vi "LabviewDemo.vi"() -> ()   [LabVIEW 2023]
uses:
  vmmsolib/vmmsolib.lvlib
panel:
  out "Support Samples":u32[](array[numeric])
  out "InitDll Return":i32
  out "Device is OK?":i32
  out "FinishDll Return":i32
  out "Voltage Wave":dbl[](graph)
  out "Voltage Array":dbl[](array[numeric]) caption="采集电压数组"
  out "ReadVoltageData Return":u32
  in  "Stop":bool
  out "Capture Return":i32
  out "Sample Success？":i32
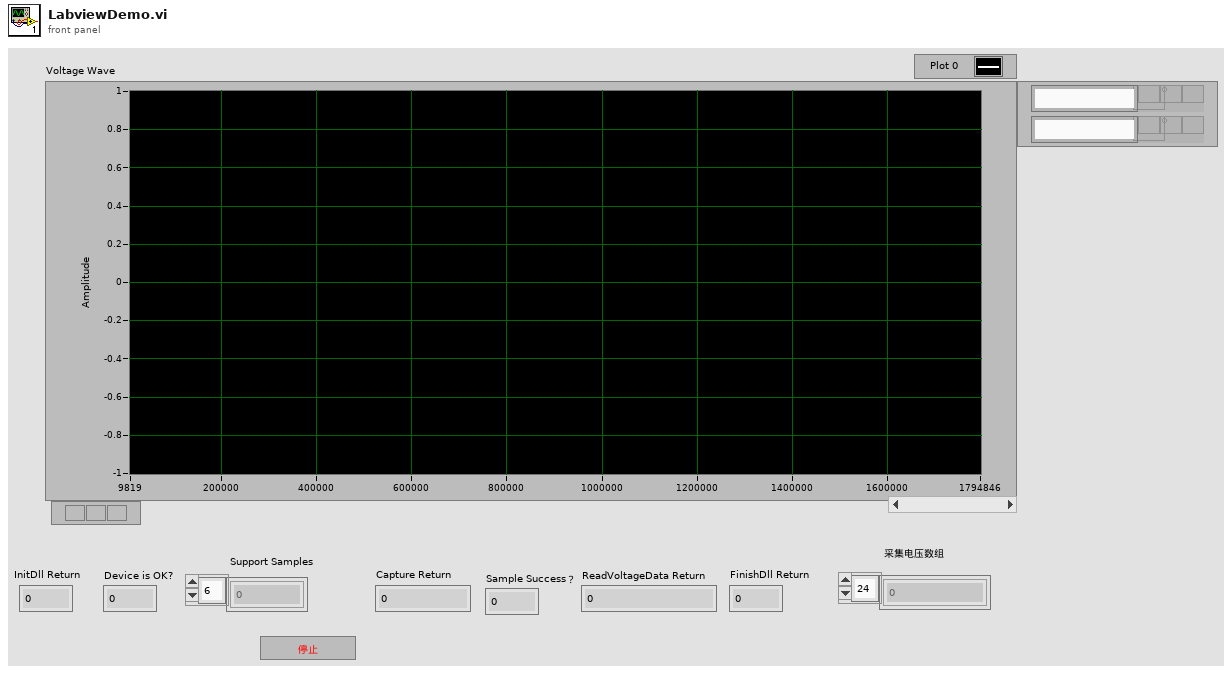
[diagram p1: front panel]
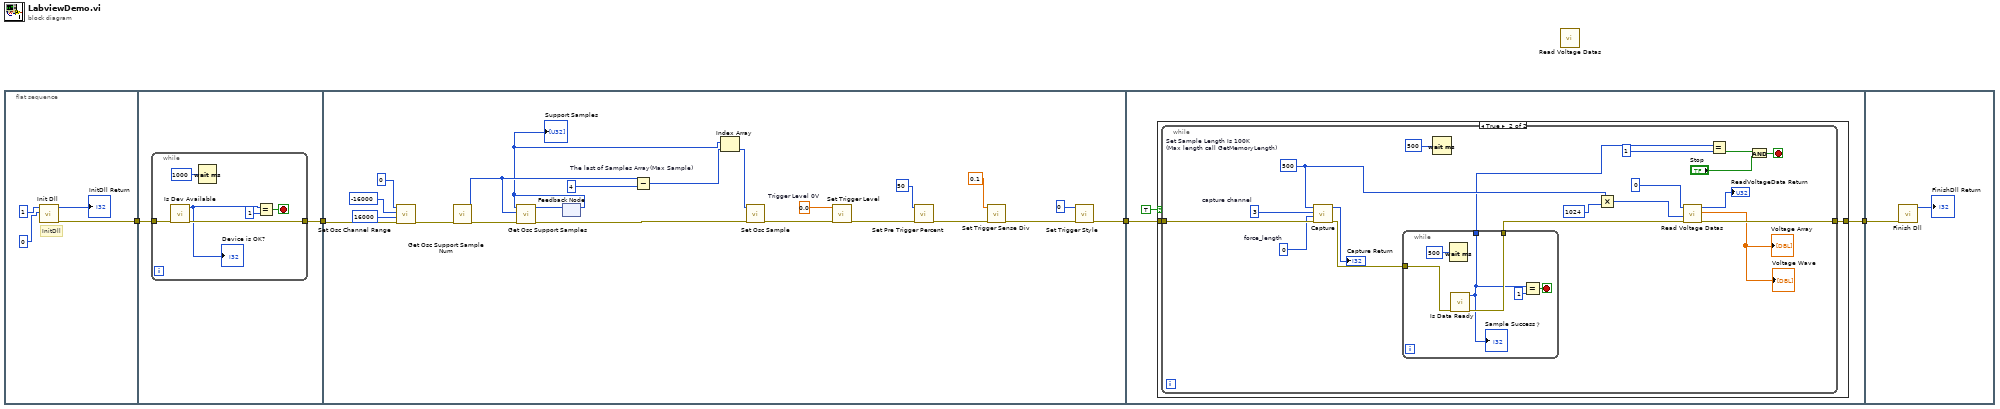
[diagram p0: block diagram]
diagram:
  n1 = flat-sequence {
    tunnel: [w8] -> w4
    tunnel: w4 -> [w10]
    tunnel: [w9] -> w3
    tunnel: w3 -> [w36]
    tunnel: [w28] -> w2
    tunnel: w2 -> [w41]
    tunnel: [w39] -> w1
    tunnel: w1 -> [w70]
    frame #0 {
      # "InitDll"
      n2 = call "Init Dll.vi"("en_hard_watchdog"=0 ("channel"), "en_log"=1 ("channel")) -> ("error out"=w8:errorcluster, "function return"=→"InitDll Return":i32)  [unwired: 8 in]
    }
    frame #1 {
      n3 = while {
        tunnel: w10 -> [w13]
        tunnel: [w12] -> w9
        stop <- w14 stop-if-true
        n4 = call "Is Dev Available.vi"("error in (no error)"=w13) -> ("error out"=w12:errorcluster, "function return"=w11:i32)  [unwired: 9 in]
        "Device is OK?" <- w11
        n5 = Wait (ms)(milliseconds to wait=u32 1000 ("等待时间（毫秒）")) -> ()  [unwired: 1 out]
        n6 = Equal?(x=w11, y=1) -> (x = y?=w14:bool)
      }
    }
    frame #2 {
      w26 = sgl 0.0  # Trigger Level 0V
      n7 = call "Set Osc Channel Range.vi"("error in (no error)"=w36, "maxmv"=16000 ("minmv"), "minmv"=-16000, "channel"=0) -> ("error out"=w25:errorcluster)  [unwired: 6 in, 1 out]
      n8 = call "Get Osc Support Sample Num.vi"("error in (no error)"=w25) -> ("error out"=w24:errorcluster, "function return"=w19:i32)  [unwired: 9 in]
      n9 = feedback #1() -> (w17:u32[])  [unwired: 1 in]
      "Support Samples" <- w17
      n10 = call "Get Osc Support Samples.vi"("error in (no error)"=w24, "maxnum"=w19, "sample"=w17) -> ("error out"=w23:errorcluster, "sample out"=w18:u32[])  [unwired: 6 in, 1 out]
      n11 = feedback-in #1(w18) -> ()
      n12 = Subtract "The last of Samples Array(Max Sample)"(x=w19, y=4 ("front")) -> (x-y=w21:i32)
      n13 = Index Array(array=w17, index=w21) -> (element=w22:u32)
      n14 = call "Set Osc Sample.vi"("error in (no error)"=w23, "sample"=w22) -> ("error out"=w33:errorcluster)  [unwired: 8 in, 1 out]
      n15 = call "Set Trigger Level.vi"("error in (no error)"=w33, "level"=w26) -> ("error out"=w31:errorcluster)  [unwired: 9 in]
      n16 = call "Set Pre Trigger Percent.vi"("error in (no error)"=w31, "front"=50) -> ("error out"=w30:errorcluster)  [unwired: 9 in]
      n17 = call "Set Trigger Sense Div.vi"("error in (no error)"=w30, "sense"=0.1) -> ("error out"=w29:errorcluster)  [unwired: 9 in]
      n18 = call "Set Trigger Style.vi"("error in (no error)"=w29, "style"=u32 0) -> ("error out"=w28:errorcluster)  [unwired: 9 in]
    }
    frame #3 {
      n19 = case shown="True" TRUE {
        tunnel: w41 -> [_ w42]
        tunnel: [_ w43] -> w39
        frame False {
        }
        frame True {
          n20 = while {
            tunnel: [w55] -> w43
            tunnel: w42 -> [w56]
            stop <- w59 stop-if-true
            w47 = i8 0  # force_length
            w52 = u32 500  # Set Sample Length Is 100K (Max length call GetMemoryLength)
            w48 = i8 3  # capture channel
            n21 = call "Capture.vi"("error in (no error)"=w56, "force_length"=w47, "capture_channel"=w48, "length"=w52) -> ("error out"=w46:errorcluster, "function return"=→"Capture Return":i32)  [unwired: 6 in]
            n22 = while {
              tunnel: w46 -> [w65]
              tunnel: [w64] -> w45
              tunnel: [w63] -> w44
              stop <- w66 stop-if-true
              n23 = Wait (ms)(milliseconds to wait=u32 500 ("等待时间（毫秒）")) -> ()  [unwired: 1 out]
              n24 = call "Is Data Ready.vi"("error in (no error)"=w65) -> ("error out"=w64:errorcluster, "function return"=w63:i32)  [unwired: 9 in]
              "Sample Success？" <- w63
              n25 = Equal?(x=w63, y=1) -> (x = y?=w66:bool)
            }
            n26 = Wait (ms)(milliseconds to wait=u32 500 ("等待时间（毫秒）")) -> ()  [unwired: 1 out]
            n27 = Multiply(x=w52, y=1024) -> (x*y=w51:u32)
            n28 = call "Read Voltage Datas.vi"("error in (no error)"=w45, "length"=w51, "channel"=i8 0) -> ("error out"=w55:errorcluster, "buffer out"=→"Voltage Array" →"Voltage Wave":dbl[], "function return"=→"ReadVoltageData Return":u32)  [unwired: 6 in]
            n29 = Equal?(x=w44, y=1) -> (x = y?=w57:bool)
            n30 = And(x=w57, y="Stop") -> (x .and. y?=w59:bool)
          }
        }
      }
    }
    frame #4 {
      n31 = call "Finish Dll.vi"("error in (no error)"=w70) -> ("function return"=→"FinishDll Return":i32)  [unwired: 9 in, 1 out]
    }
  }
  n32 = call "Read Voltage Datas.vi"() -> ()  [unwired: 9 in, 3 out]
